vi "Display Format.vi"(8 "error in":errorcluster, 11 "Surface Pointer":u32) -> (0 "error out":errorcluster, 3 "Surface Pointer":u32)   [LabVIEW 2014, in "LibSDL2.lvlib"]
uses:
  LibSDL2.lvlib
  DLL/SDL2.dll
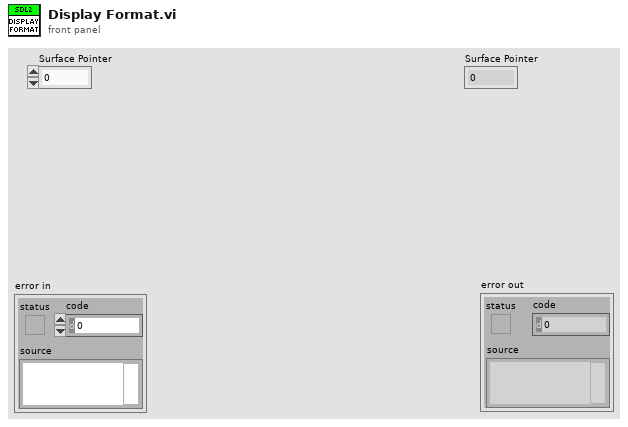
[diagram p1: front panel]
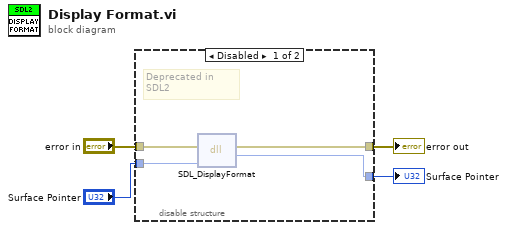
[diagram p0: block diagram]
diagram:
  n1 = disable-structure shown="Disabled" {
    disable-tunnel: "error in" -> [w8 _]
    disable-tunnel: "Surface Pointer" -> [w7 _]
    disable-tunnel: [w6 _] -> w2
    disable-tunnel: [w5 _] -> w1
    frame Disabled {
      # "Deprecated in SDL2"
      n2 = dll-call lib="C:/dev/PGS/LabSDL2/Source/LibSDL2 Wrapper/DLL/SDL2.dll" fn="SDL_DisplayFormat"(error in=w8, "surface"=w7) -> (error out=w6:errorcluster, "return type"=w5:u32)  [unwired: 3 in, 1 out]
    }
    frame Enabled {
    }
  }
  "error out" <- w2
  "Surface Pointer" <- w1
